vi "Waveforms Generation RT Driver VI.vi"(6 "Device Clock":string, 9 "Device Inputs FIFO":refnum<k33>, 10 "Device Outputs FIFO":refnum<k33>, 11 "Device Reference":T1 format="%.0x") -> ()   [LabVIEW 2013, in "Waveforms Generation Custom Device.lvlib"]
uses:
  Waveforms Generation Custom Device.lvlib
  <vilib>/NI Veristand/Custom Device API/Custom Device Item Ref.ctl
  RT state data.ctl
  <vilib>/NI Veristand/Custom Device API/Waveform Data Reference.ctl
  <vilib>/NI Veristand/Custom Device Waveform API/Multiple Waveforms Write (DBL)/Multiple Waveforms Write (DBL).lvclass
  <vilib>/NI Veristand/Custom Device API/Custom Device Channel Type.ctl
  <vilib>/NI Veristand/Custom Device Waveform API/Communication Properties.ctl
  <vilib>/NI Veristand/Custom Device Waveform API/Waveform Session.lvclass/Waveform Session.ctl
  <vilib>/NI Veristand/Custom Device Waveform API/Multiple Waveforms Write (DBL)/Multiple Waveforms Write (DBL).lvclass/Multiple Waveforms Write (DBL).ctl
  <vilib>/NI Veristand/Custom Device Waveform API/Internal Comm Classes/WPL Comm/WPL Comm.lvclass/WPL Comm.ctl
  <vilib>/NI Veristand/Custom Device Waveform API/Internal Comm Classes/WPL Comm/WPL Comm (2D DBL)/WPL Comm (2D DBL).lvclass/WPL Comm (2D DBL).ctl
  Open waveform write sessions.vi
  <vilib>/NI Veristand/Custom Device Waveform API/NI VeriStand - Write Waveform(s).vi
  <vilib>/NI Veristand/Custom Device Waveform API/Multiple Waveforms Write (DBL)/NI VeriStand - Write Multiple Waveforms (DBL).vi
  <vilib>/NI Veristand/Custom Device Waveform API/NI VeriStand - Start Waveform(s).vi
  <vilib>/NI Veristand/Custom Device Waveform API/Multiple Waveforms Write (DBL)/NI VeriStand - Start Multiple Waveforms (DBL).vi
  <vilib>/NI Veristand/Custom Device Waveform API/Read Sample offset DVR.vi
  <vilib>/NI Veristand/Custom Device Waveform API/Internal Comm Classes/WPL Comm/WPL Comm (2D DBL)/Comm_write 2d dbl.vi
  <vilib>/NI Veristand/Custom Device Waveform API/Check Write Size.vi
  <vilib>/NI Veristand/Custom Device Waveform API/Check Opened.vi
  <vilib>/NI Veristand/Custom Device Waveform API/Internal Comm Classes/WPL Comm/WPL_start dbl waveform.vi
  <vilib>/NI Veristand/Custom Device Waveform API/Internal Comm Classes/WPL Comm/Direct Send WPL Command.vi
  <vilib>/NI Veristand/Custom Device Waveform API/Internal Comm Classes/WPL Comm/Convert Q Error to Shutdown Error.vi
  <vilib>/NI Veristand/Custom Device Waveform API/Internal Comm Classes/WPL Comm/Set t0 on Variant.vi
  <vilib>/NI Veristand/Custom Device Waveform API/Internal Comm Classes/WPL Comm/Send WPL Command.vi
  <vilib>/NI Veristand/Custom Device Waveform API/Multiple Waveforms Write (DBL)/NI VeriStand - Open Multiple Waveforms Write Session (DBL).vi
  <vilib>/NI Veristand/Custom Device API/Get Item Property (Double).vi
  <userlib>/_OpenG.lib/error/error.llb/Filter Error Codes (Array)__ogtk.vi
  <vilib>/Utility/error.llb/Error Cluster From Error Code.vi
  <vilib>/measure/masignal.llb/Basic Function Generator.vi
  <vilib>/NI Veristand/Custom Device Waveform API/Multiple Waveforms Write (DBL)/NI VeriStand - Close Multiple Waveforms Write Session (DBL).vi
  <vilib>/NI VeriStand/Custom Device Tools/Custom Device Utility Library/Custom Device Utility Library.lvlib
  <vilib>/NI Veristand/Custom Device API/Custom Device API.lvlib
  <vilib>/NI Veristand/Custom Device API/Message Response (String).ctl
  <vilib>/NI Veristand/Custom Device API/Message Response (Byte Array).ctl
  <vilib>/NI Veristand/Custom Device Waveform API/NI_VS Custom Device Waveform API.lvlib
panel:
  in  "Initialization Status Notifier":refnum<notifier>
  in  "Status Notifier":refnum<notifier>
  # "Custom Device Template\nv1.0"
  # "Use this template as a starting point for creating a custom device code module. The input controls shown here are specially named controls that the system will use to provide the device loop with data. The controls are not required for the device loop to run. For instance, if the device doesn't produce any output data, then you don't need the Device Outputs FIFO control. If you do use these controls, however, they need to have these exact names to be functional."
  # "The optional status notifier element is used to notify the RT engine of the last state of the custom device, and to indicate the device has completed execution. If this control is not used, a default No Error value is returned to the system when the device finishes execution.\n\nNote: This error state is not checked until the system shuts down. Use an output status channel to send more immediate status values to the system."
  # "This optional input can be used to send the VeriStand Engine the final status of the custom device initalization process. If this control exists on the custom device front panel, the VeriStand Engine will wait for a status update before starting up. If the custom device reports an error, that will abort the execution of the current configuration in the VeriStand Engine.\n\nThis control can be deleted if the custom device does not need to send the initialization status update."
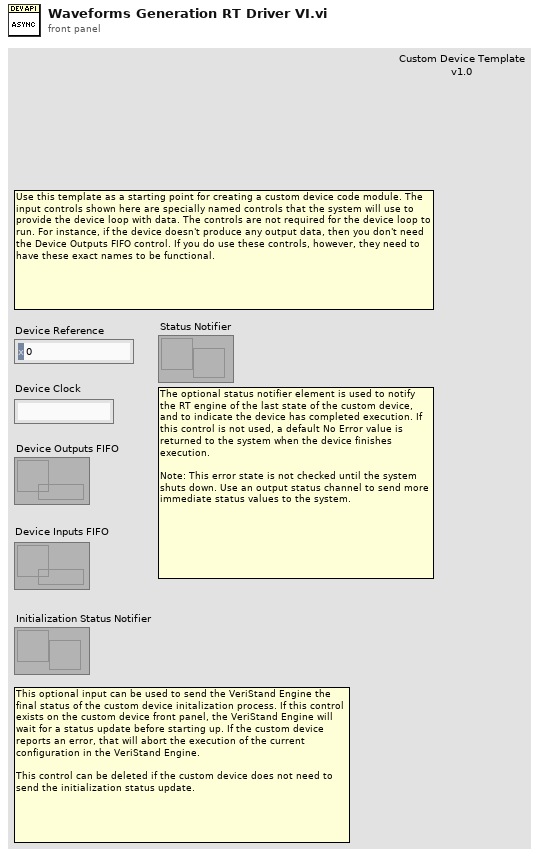
[diagram p1: front panel]
types:
  T1 = typedef "Custom Device API.lvlib/Custom Device Item Ref.ctl" = u64
  T2 = typedef "NI_VS Custom Device Waveform API.lvlib/Communication Properties.ctl" = cluster{"WPL":cluster{"Custom Queue Size":i32, "Use Custom Queue Size?":bool}}
  T3 = typedef "Custom Device API.lvlib/Custom Device Channel Type.ctl" = enum16{"Input", "Output"}
  T4 = typedef "Waveforms Generation Custom Device.lvlib/RT state data.ctl" = cluster{"Device Outputs FIFO":refnum<k33>, "Device Inputs FIFO":refnum<k33>, "ChannelOuputs":dbl[], "ChannelInputs":dbl[], "WriteSessionStarted?":bool, "Write Refs":T5[], "Multiple Waveforms Write Session (DBL)":refnum<class "Multiple Waveforms Write (DBL).lvclass">}
  T5 = typedef "Custom Device API.lvlib/Waveform Data Reference.ctl" = i32
  T6 = typedef "Custom Device API.lvlib/Custom Device Engine Event Ref.ctl" = refnum<event-registration>
  T7 = typedef "Custom Device API.lvlib/Message Response (String).ctl" = cluster{"Response":string, "Error":errorcluster}
  T8 = typedef "Custom Device API.lvlib/Message Response (Byte Array).ctl" = cluster{"Response":u8[], "Error":errorcluster}
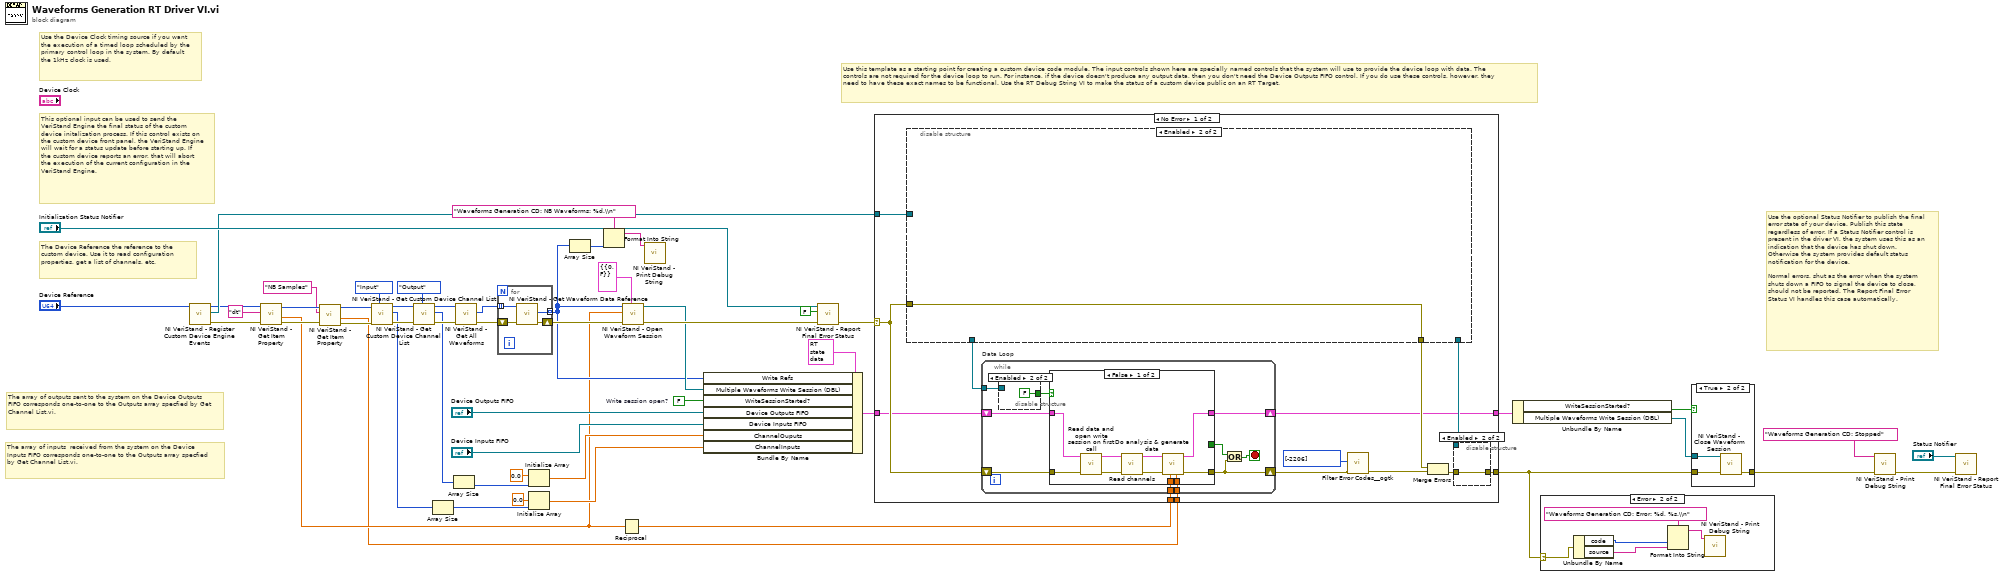
[diagram p0: block diagram]
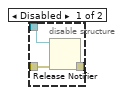
[diagram p4: hidden frame]
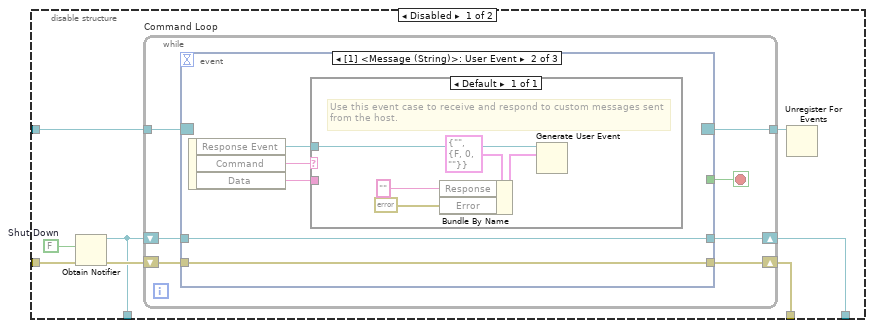
[diagram p5: hidden frame]
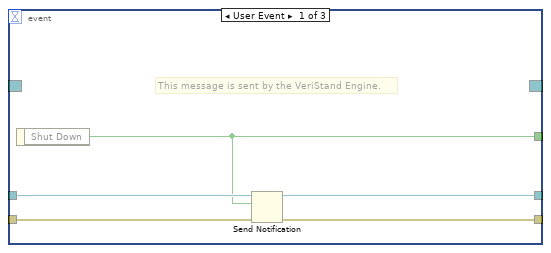
[diagram p6: hidden frame]
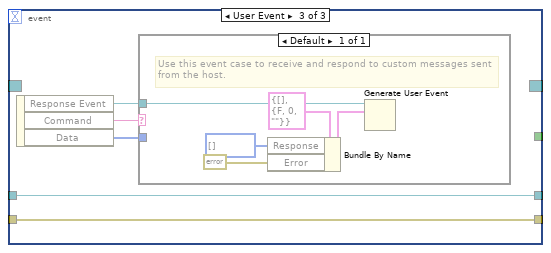
[diagram p7: hidden frame]
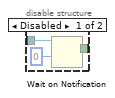
[diagram p8: hidden frame]
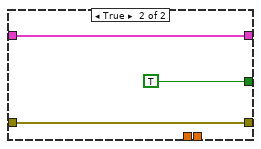
[diagram p9: hidden frame]
diagram:
  w42 = FALSE  # Write session open?
  # "This optional input can be used to send the VeriStand Engine the final status of the custom device initalization process. If this control exists on the custom device front panel, the VeriStand Engine will wait for a status update before starting up. If the custom device reports an error, that will abort the execution of the current configuration in the VeriStand Engine."
  # "The array of inputs  received from the system on the Device Inputs FIFO corresponds one-to-one to the Outputs array specfied by Get Channel List.vi."
  # "Use the optional Status Notifier to publish the final error state of your device. Publish this state regardless of error. If a Status Notifier control is present in the driver VI, the system uses this as an indication that the device has shut down. Otherwise the system provides default status notification for the device.\n\nNormal errors, shut as the error when the system shuts down a FIFO to signal the device to close, should not be reported. The Report Final Error Status VI handles this case automatically."
  # "The array of outputs sent to the system on the Device Outputs FIFO corresponds one-to-one to the Outputs array specfied by Get Channel List.vi."
  # "The Device Reference the reference to the custom device. Use it to read configuration properties, get a list of channels, etc."
  # "Use the Device Clock timing source if you want the execution of a timed loop scheduled by the primary control loop in the system. By default the 1kHz clock is used."
  # "Use this template as a starting point for creating a custom device code module. The input controls shown here are specially named controls that the system will use to provide the device loop with data. The controls are not required for the device loop to run. For instance, if the device doesn't produce any output data, then you don't need the Device Outputs FIFO control. If you do use these controls, however, they need to have these exact names to be functional. Use the RT Debug String VI to make the status of a custom device public on an RT Target."
  n1 = call <vilib>:"NI VeriStand - Register Custom Device Engine Events.vi"("Device Ref in"="Device Reference") -> ("error out"=w6:errorcluster, "Custom Device Engine Event Ref"=w51:T6, "Device Ref out"=w9:T1)  [unwired: 8 in]
  n2 = call-poly <vilib>:"NI VeriStand - Get Item Property.vi"("error in (no error)"=w6, "Property Name"="dt", "Item Ref in"=w9) -> ("error out"=w12:errorcluster, "Value"=w5:dbl, "Item Ref out"=w11:T1)  [unwired: 5 in, 1 out]
  n3 = call-poly <vilib>:"NI VeriStand - Get Item Property.vi"("error in (no error)"=w12, "Property Name"="NB Samples", "Item Ref in"=w11) -> ("error out"=w7:errorcluster, "Value"=w4:dbl, "Item Ref out"=w8:T1)  [unwired: 5 in, 1 out]
  n4 = call <vilib>:"NI VeriStand - Get Custom Device Channel List.vi"("Channel Type"=Custom_Device_Channel_Type."Input", "error in (no error)"=w7, "Device Ref in"=w8) -> ("error out"=w30:errorcluster, "Specified Channel Ref List"=w25:T1[], "Device Ref out"=w29:T1)  [unwired: 6 in]
  n5 = call <vilib>:"NI VeriStand - Get Custom Device Channel List.vi"("Channel Type"=Custom_Device_Channel_Type."Output", "error in (no error)"=w30, "Device Ref in"=w29) -> ("error out"=w28:errorcluster, "Specified Channel Ref List"=w22:T1[], "Device Ref out"=w27:T1)  [unwired: 6 in]
  n6 = Array Size(array=w25) -> (size(s)=w24:i32)
  n7 = Array Size(array=w22) -> (size(s)=w21:i32)
  n8 = call <vilib>:"NI VeriStand - Get All Waveforms.vi"("error in"=w28, "Section Ref in"=w27) -> ("error out"=w32:errorcluster, "Waveform Refs"=w33:T1[])  [unwired: 6 in, 2 out]
  n9 = for {
    shift-right: [w56] -> w47
    shift-left: w32 -> [w57]
    tunnel: w33 -> [w55] mode=indexing
    tunnel: [w54] -> w19 mode=indexing
    n10 = call <vilib>:"NI VeriStand - Get Waveform Data Reference.vi"("error in (no error)"=w57, "Waveform Ref in"=w55) -> ("error out"=w56:errorcluster, "Waveform Data Reference"=w54:T5)  [unwired: 7 in, 1 out]
  }
  n11 = Initialize Array(0.0 ("element"), w21) -> (w39:dbl[])
  n12 = Initialize Array(0.0 ("element"), w24) -> (w38:dbl[])
  n13 = Array Size(array=w19) -> (size(s)=w18:i32)
  n14 = Format Into String(format string="Waveforms Generation CD: NB Waveforms: %d.\\n", w18) -> (resulting string=w17:string)  [unwired: 2 in, 1 out]
  n15 = Reciprocal(x=w5) -> (1/x=w20:dbl)
  n16 = call-poly <vilib>:"NI VeriStand - Open Waveform Session.vi"("Communication Properties"=T2 {"WPL"={"Custom Queue Size"=0, "Use Custom Queue Size?"=FALSE}}, "error in (no error)"=w47, "dt"=w5, "DBL Waveform Data References"=w19) -> ("error out"=w46:errorcluster, "Multiple Waveforms Write Session (DBL)"=w31:refnum<class "Multiple Waveforms Write (DBL).lvclass">)  [unwired: 6 in]
  n17 = call <vilib>:"NI VeriStand - Print Debug String.vi"("Message"=w17) -> ()  [unwired: 10 in, 1 out]
  n18 = Bundle By Name(cluster=T4 {"Device Outputs FIFO"=refnum, "Device Inputs FIFO"=refnum, "ChannelOuputs"=[], "ChannelInputs"=[], "WriteSessionStarted?"=FALSE, "Write Refs"=[], "Multiple Waveforms Write Session (DBL)"=refnum} ("RT State Data"), "Write Refs"=w19, "Multiple Waveforms Write Session (DBL)"=w31, "WriteSessionStarted?"=w42, "Device Outputs FIFO"="Device Outputs FIFO", "Device Inputs FIFO"="Device Inputs FIFO", "ChannelOuputs"=w39, "ChannelInputs"=w38) -> (w37:T4)
  n19 = call <vilib>:"NI VeriStand - Report Final Error Status.vi"("error in (no error)"=w46, "Filter FIFO & Shutdown Errors (T)"=FALSE ("Filter FIFO Errors (T)"), "Status Notifier"="Initialization Status Notifier") -> ("error out"=w49:errorcluster)  [unwired: 8 out]
  n20 = case shown="No Error" w49 {
    selector: w49 -> [w67 w145]
    tunnel: w51 -> [w71 _]
    tunnel: [w70 w145] -> w14
    tunnel: w37 -> [w64 w144]
    tunnel: [w63 w144] -> w36
    tunnel: w20 -> [w62 _]
    tunnel: w4 -> [w58 _]
    frame No Error {
      n21 = disable-structure shown="Enabled" {
        disable-tunnel: w71 -> [w82 _]
        disable-tunnel: [w79 _] -> w69
        disable-tunnel: [w78 _] -> w68
        disable-tunnel: w67 -> [w77 w116]
        disable-tunnel: [w76 w116] -> w65
        frame Disabled {
          w81 = FALSE  # Shut Down
          n22 = Obtain Notifier(notification data type=w81, error in (no error)=w77) -> (notifier out=w79:refnum<notifier>, error out=w83:errorcluster)  [unwired: 2 in, 1 out]
          n23 = while "Command Loop" {
            tunnel: w82 -> [w90]
            tunnel: [w89] -> w80
            shift-right: [w86] -> w78
            shift-left: w79 -> [w87]
            shift-right: [w84] -> w76
            shift-left: w83 -> [w85]
            stop <- w88 stop-if-true
            n24 = event shown="[1] <Message (String)>: User Event" {
              selector: w90 -> [_ _ _]
              dyn-events: [_ _ _] -> w89
              timeout: _ -> [_ _ _]
              tunnel: [w93 _ _] -> w88
              tunnel: w87 -> [w94 w98 w108]
              tunnel: [w95 w98 w108] -> w86
              tunnel: w85 -> [w92 w96 w106]
              tunnel: [w91 w96 w106] -> w84
              event User Event {
                # "This message is sent by the VeriStand Engine."
                n25 = event-data() -> ("Shut Down"=w93:bool)  [unwired: 1 in]
                n26 = Send Notification(notification=w93, notifier=w94, error in (no error)=w92) -> (notifier out=w95:refnum<notifier>, error out=w91:errorcluster)
              }
              event User Event {
                n27 = event-data() -> ("Response Event"=w97:refnum<user-event>, "Command"=w100:string, "Data"=w99:string)  [unwired: 1 in]
                n28 = case shown="Default" w100 {
                  tunnel: w99 -> [_]
                  tunnel: w97 -> [w105]
                  frame Default {
                    # "Use this event case to receive and respond to custom messages sent from the host."
                    n29 = Bundle By Name(cluster=T7 {"Response"="", "Error"={"status"=FALSE, "code"=0, "source"=""}} ("event data"), "Response"="", "Error"=errorcluster {"status"=FALSE, "code"=0, "source"=""}) -> (w103:T7)
                    n30 = Generate User Event(user event=w105, event data cluster=w103) -> ()  [unwired: 2 in, 2 out]
                  }
                }
              }
              event User Event {
                n31 = event-data() -> ("Response Event"=w107:refnum<user-event>, "Command"=w110:string, "Data"=w109:u8[])  [unwired: 1 in]
                n32 = case shown="Default" w110 {
                  tunnel: w109 -> [_]
                  tunnel: w107 -> [w115]
                  frame Default {
                    # "Use this event case to receive and respond to custom messages sent from the host."
                    n33 = Bundle By Name(cluster=T8 {"Response"=[], "Error"={"status"=FALSE, "code"=0, "source"=""}} ("event data"), "Response"=u8[] [], "Error"=errorcluster {"status"=FALSE, "code"=0, "source"=""}) -> (w112:T8)
                    n34 = Generate User Event(user event=w115, event data cluster=w112) -> ()  [unwired: 2 in, 2 out]
                  }
                }
              }
            }
          }
          n35 = Unregister For Events(event registration refnum=w80) -> ()  [unwired: 1 in, 1 out]
        }
        frame Enabled {
        }
      }
      n36 = while "Data Loop" {
        shift-right: [w121] -> w61
        shift-left: w67 -> [w126]
        tunnel: w69 -> [w125]
        shift-right: [w119] -> w63
        shift-left: w64 -> [w120]
        tunnel: w62 -> [w118]
        tunnel: w58 -> [w117]
        stop <- w122 stop-if-true
        n37 = disable-structure shown="Enabled" {
          disable-tunnel: w125 -> [w128 _]
          disable-tunnel: [w127 FALSE ("Shut Down")] -> w124
          frame Disabled {
            n38 = Wait on Notification(notifier=w128, timeout in ms (-1)=0) -> (notification=w127:bool)  [unwired: 2 in, 3 out]
          }
          frame Enabled {
          }
        }
        n39 = case shown="False" w124 {
          tunnel: w126 -> [w140 w143]
          tunnel: [w137 w143] -> w121
          tunnel: [_ TRUE] -> w123
          tunnel: w120 -> [w139 w141]
          tunnel: [w138 w141] -> w119
          tunnel: w118 -> [w132 _]
          tunnel: w117 -> [w131 _]
          frame False {
            n40 = call "Read data and open write session on first call.vi"("error in (no error)"=w140, "RT State Data in"=w139) -> ("error out"=w136:errorcluster, "RT State Data out"=w135:T4)  [unwired: 8 in]
            n41 = call "Read channels.vi"("error in (no error)"=w136, "RT State Data in"=w135) -> ("error out"=w133:errorcluster, "RT State Data out"=w134:T4)  [unwired: 8 in]
            n42 = call "Do analysis & generate data.vi"("NB Samples"=w131, "Sample Frequency (S/s)"=w132, "error in (no error)"=w133, "RT State Data in"=w134) -> ("error out"=w137:errorcluster, "RT State Data out"=w138:T4)  [unwired: 6 in]
          }
          frame True {
          }
        }
        n43 = Or(x=w123, y=w121) -> (x .or. y?=w122:bool)
      }
      n44 = call-poly <userlib>:"Filter Error Codes__ogtk.vi"("Error In"=w61, "Error Codes to Filter"=i32[] [-2206]) -> ("Error Out"=w60:errorcluster)  [unwired: 7 in, 2 out]
      n45 = Merge Errors(w65, w60) -> (w66:errorcluster)
      n46 = disable-structure shown="Enabled" {
        disable-tunnel: [w74 w75] -> w70
        disable-tunnel: w68 -> [w73 _]
        disable-tunnel: w66 -> [w72 w75]
        frame Disabled {
          n47 = Release Notifier(notifier=w73, error in (no error)=w72) -> (error out=w74:errorcluster)  [unwired: 1 in, 2 out]
        }
        frame Enabled {
        }
      }
    }
    frame Error {
    }
  }
  n48 = Unbundle By Name(w36) -> ("WriteSessionStarted?"=w35:bool, "Multiple Waveforms Write Session (DBL)"=w34:refnum<class "Multiple Waveforms Write (DBL).lvclass">)
  n49 = case shown="Error" w14 {
    selector: w14 -> [_ w150]
    frame No Error {
    }
    frame Error {
      n50 = Unbundle By Name(w150) -> ("code"=w149:i32, "source"=w148:string)
      n51 = Format Into String(format string="Waveforms Generation CD: Error: %d, %s.\\n", w149, w148) -> (resulting string=w147:string)  [unwired: 2 in, 1 out]
      n52 = call <vilib>:"NI VeriStand - Print Debug String.vi"("Message"=w147) -> ()  [unwired: 10 in, 1 out]
    }
  }
  n53 = case shown="True" w35 {
    tunnel: w14 -> [w151 w153]
    tunnel: [w151 w154] -> w3
    tunnel: w34 -> [_ w152]
    frame False {
    }
    frame True {
      n54 = call-poly <vilib>:"NI VeriStand - Close Waveform Session.vi"("error in (no error)"=w153, "Multiple Waveforms Write Session (DBL)"=w152) -> ("error out"=w154:errorcluster)  [unwired: 9 in]
    }
  }
  n55 = call <vilib>:"NI VeriStand - Print Debug String.vi"("error in (no error)"=w3, "Message"="Waveforms Generation CD: Stopped") -> ("error out"=w2:errorcluster)  [unwired: 9 in]
  n56 = call <vilib>:"NI VeriStand - Report Final Error Status.vi"("error in (no error)"=w2, "Status Notifier"="Status Notifier") -> ()  [unwired: 1 in, 9 out]
